vi "editConfigurationMain.vi"(8 "error in (no error)":errorcluster, 11 "ConfigurationTabUI in":refnum<class "ConfigurationTabUI.lvclass">) -> (0 "error out":errorcluster, 3 "ConfigurationTabUI out":refnum<class "ConfigurationTabUI.lvclass">)   [LabVIEW 2015, in "ExampleConfiguration.lvlib" / "ConfigurationTabUI.lvclass"]
doc: "Starts the configuration editor."
uses:
  ConfigurationTabUI.lvclass
  ComponentTemplateCore/ConfigurationWithXML/MyComputer/Configuration/ConfigurationTabUI/ConfigurationTabUI.lvclass
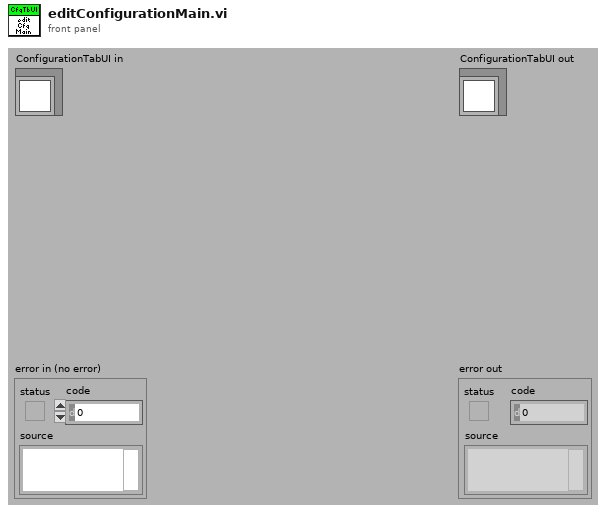
[diagram p1: front panel]
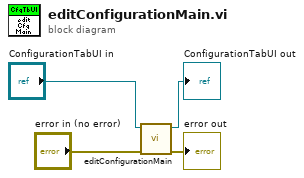
[diagram p0: block diagram]
diagram:
  n1 = call-parent "editConfigurationMain.vi"("error in (no error)"="error in (no error)", "ConfigurationTabUI in"="ConfigurationTabUI in") -> ("error out"=→"error out":errorcluster, "ConfigurationTabUI out"=→"ConfigurationTabUI out":refnum<class "ConfigurationTabUI.lvclass">)  [unwired: 8 in]
